vi "RTS Check First Door Ops Cycle.vi"(5 "Door Open Sequence:":T5, 7 "Array Size":i32, 8 "error in (no error)":errorcluster, 11 "Station 1-8 Data in":T1 {"Station Slide"."Chamber 1-1"."Start Time" format="%<%X\n%x>T"; "Station Slide"."Chamber 1-1"."End Time" format="%<%X\n%x>T"; "Station Slide"."Time Count (s)" format="%.2f"; "Station Cab"."Chamber 1-1"."Start Time" format="%<%X\n%x>T"; "Station Cab"."Chamber 1-1"."End Time" format="%<%X\n%x>T"; "Station Cab"."Time Count (s)" format="%.2f"; "Station Freezer"."Chamber 1-1"."Start Time" format="%<%X\n%x>T"; "Station Freezer"."Chamber 1-1"."End Time" format="%<%X\n%x>T"; "Station Freezer"."Time Count (s)" format="%.2f"}) -> (0 "error out":errorcluster, 3 "First Cycle Complete":bool)   [LabVIEW 2016]
uses:
  Type Definitions/RTS Door Ops Sequence.ctl
  Type Definitions/RTS Station Relay Ops.ctl
  Type Definitions/RTS Door Opener Indicator.ctl
  Type Definitions/RTS Door Ops Client.ctl
  Type Definitions/RTS Door Opening Schedule.ctl
panel:
  # "Chamber Conditions:"
  # "Chamber Conditions:"
  # "Chamber Conditions:"
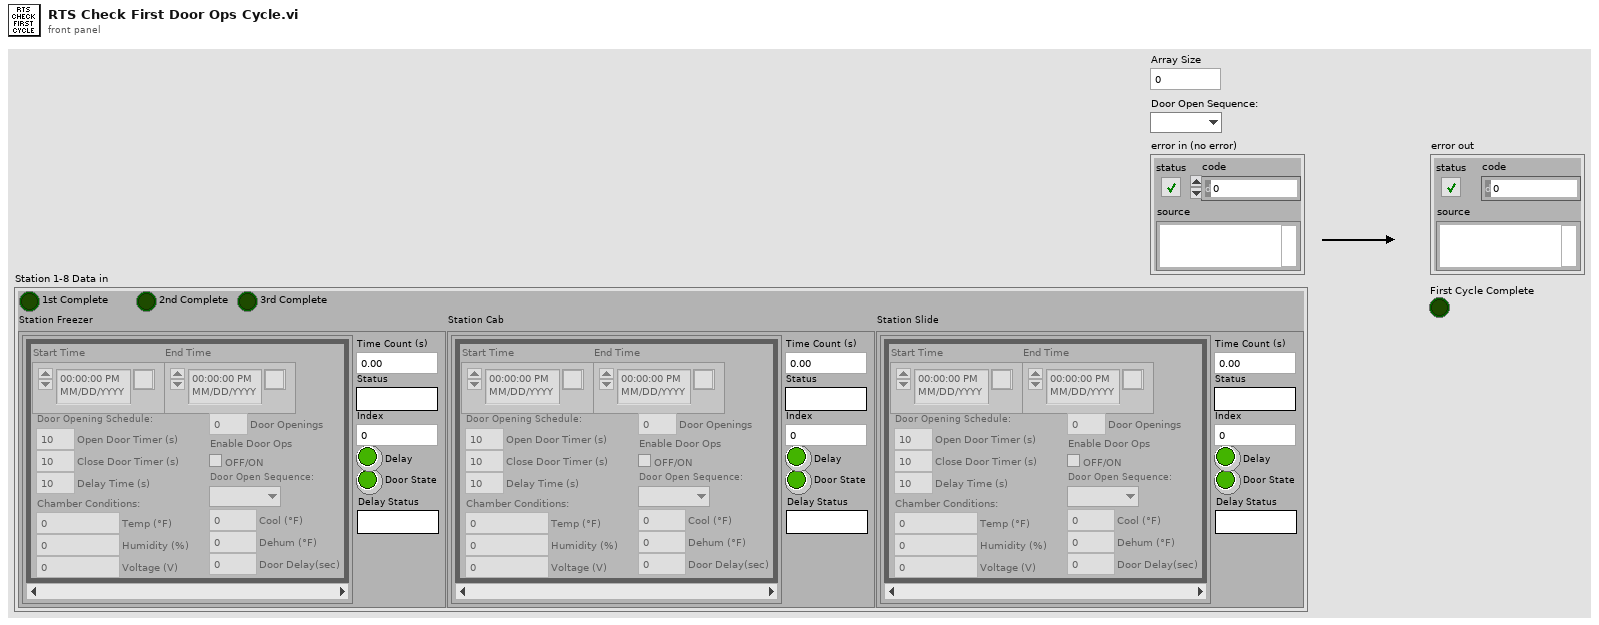
[diagram p1: front panel]
types:
  T1 = typedef "RTS Station Relay Ops.ctl" = cluster{"Station Freezer":T2, "Station Cab":T2, "Station Slide":T2, "1st Complete":bool, "2nd Complete":bool, "3rd Complete":bool}
  T2 = typedef "RTS Door Opener Indicator.ctl" = cluster{"Time Count (s)":dbl, "Status":string, "Door State":bool, "Delay":bool, "Chamber 1-1":T3[], "Index":i32, "Delay Status":string}
  T3 = typedef "RTS Door Ops Client.ctl" = cluster{"End Time":timestamp, "Start Time":timestamp, "Door Opening Schedule:":T4, "Enable Door Ops":bool, "Door Openings":u32, "Temp (°F)":dbl, "Humidity (%)":dbl, "Voltage (V)":dbl, "Door Open Sequence:":T5, "Door Delay(sec)":dbl, "Dehum (°F)":dbl, "Cool (°F)":dbl}
  T4 = typedef "RTS Door Opening Schedule.ctl" = cluster{"Open Door Timer (s)":dbl, "Delay Time (s)":dbl, "Close Door Timer (s)":dbl}
  T5 = typedef "RTS Door Ops Sequence.ctl" = enum16{"", "1st", "2nd", "3rd"}
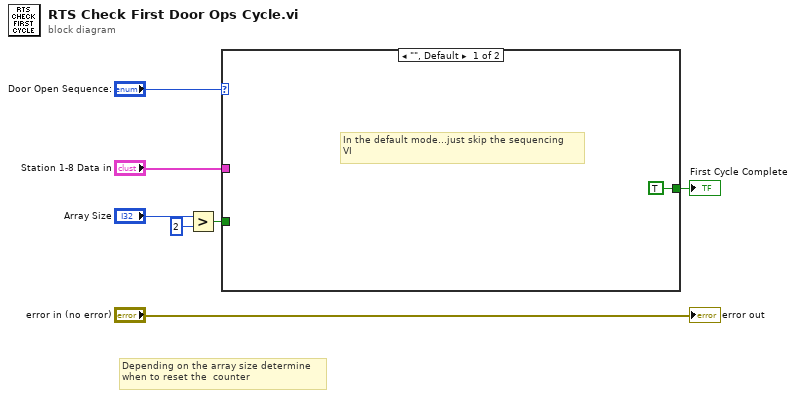
[diagram p0: block diagram]
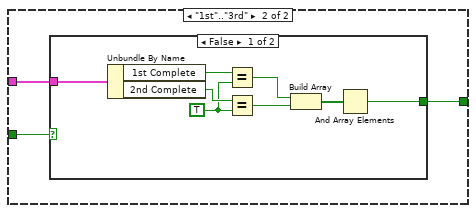
[diagram p2: hidden frame]
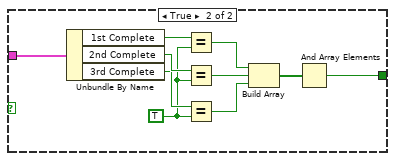
[diagram p3: hidden frame]
diagram:
  # "Depending on the array size determine\nwhen to reset the  counter"
  n1 = Greater?(x="Array Size", y=2) -> (0:w6:bool)
  n2 = case shown="\"\", Default" "Door Open Sequence:" {
    tunnel: "Station 1-8 Data in" -> [_ w10]
    tunnel: w6 -> [_ w11]
    tunnel: [TRUE w9] -> w1
    frame "", Default {
      # "In the default mode...just skip the sequencing\nVI"
    }
    frame "1st".."3rd" {
      n3 = case shown="False" w11 {
        tunnel: w10 -> [w13 w21]
        tunnel: [w12 w20] -> w9
        frame False {
          w17 = TRUE ("y")
          n4 = Unbundle By Name(w13) -> ("1st Complete"=w19:bool, "2nd Complete"=w18:bool)
          n5 = Equal?(x=w19, y=w17) -> (x = y?=w16:bool)
          n6 = Equal?(x=w18, y=w17) -> (x = y?=w15:bool)
          n7 = Build Array(w16, w15) -> (w14:bool[])
          n8 = And Array Elements(Boolean array=w14) -> (logical AND=w12:bool)
        }
        frame True {
          w26 = TRUE ("y")
          n9 = Unbundle By Name(w21) -> ("1st Complete"=w29:bool, "2nd Complete"=w28:bool, "3rd Complete"=w27:bool)
          n10 = Equal?(x=w29, y=w26) -> (x = y?=w25:bool)
          n11 = Equal?(x=w28, y=w26) -> (x = y?=w24:bool)
          n12 = Equal?(x=w27, y=w26) -> (x = y?=w23:bool)
          n13 = Build Array(w25, w24, w23) -> (w22:bool[])
          n14 = And Array Elements(Boolean array=w22) -> (logical AND=w20:bool)
        }
      }
    }
  }
  "First Cycle Complete" <- w1
  "error out" <- "error in (no error)"
